vi "Angle 0 to 360.vi"(1 "Angle in":dbl) -> (0 "Angle out":dbl)   [LabVIEW 2025]
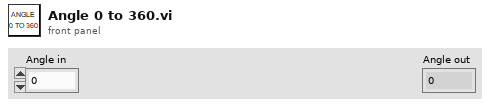
[diagram p1: front panel]
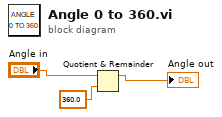
[diagram p0: block diagram]
diagram:
  n1 = Quotient & Remainder(x="Angle in", y=360.0) -> (x-y*floor(x/y)=→"Angle out":dbl)  [unwired: 1 out]
